vi "pulse data FFTfilter.vi"() -> ()   [LabVIEW 2016]
uses:
  <vilib>/Analysis/2dsp.llb/Real FFT.vi
  <vilib>/Analysis/2dsp.llb/Inverse Real FFT.vi
  <vilib>/Analysis/NI_AALPro.lvlib
panel:
  in  "lower cut off":dbl format="%.2f"
  in  "upper cut off":dbl=50000.0 format="%.2f"
  in  "filter":u16(ring) items=["Band Pass", "Band Stop"]
  in  "save interpolation?":bool
  in  "format":string="%f"
  in  "average traces?":u8=1 min=1 step=1
  in  "save plot?":bool
  in  "format":string="%f"
  out "plotted data":cluster{dbl[], dbl[]}(graph)
  in  "type of interpolation":u16(ring) items=["linear", "cubic spline", "polynomial"]
  in  "no. 1/B interpolation points":u16(ring) items=["1024", "2048", "4096", "8192", "16384", "32768"]
  in  "y domain":u16(ring) items=["channel A"]
  in  "x domain":u16(ring) items=["time (rising field)", "time (falling field)", "1/B (rising field)", "1/B (falling field)", "1/B (rising field + falling field)", "1/B (rising field - falling field)"]
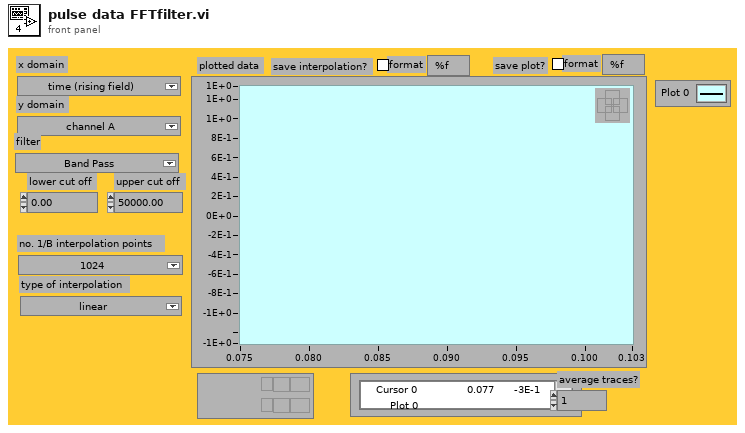
[diagram p1: front panel]
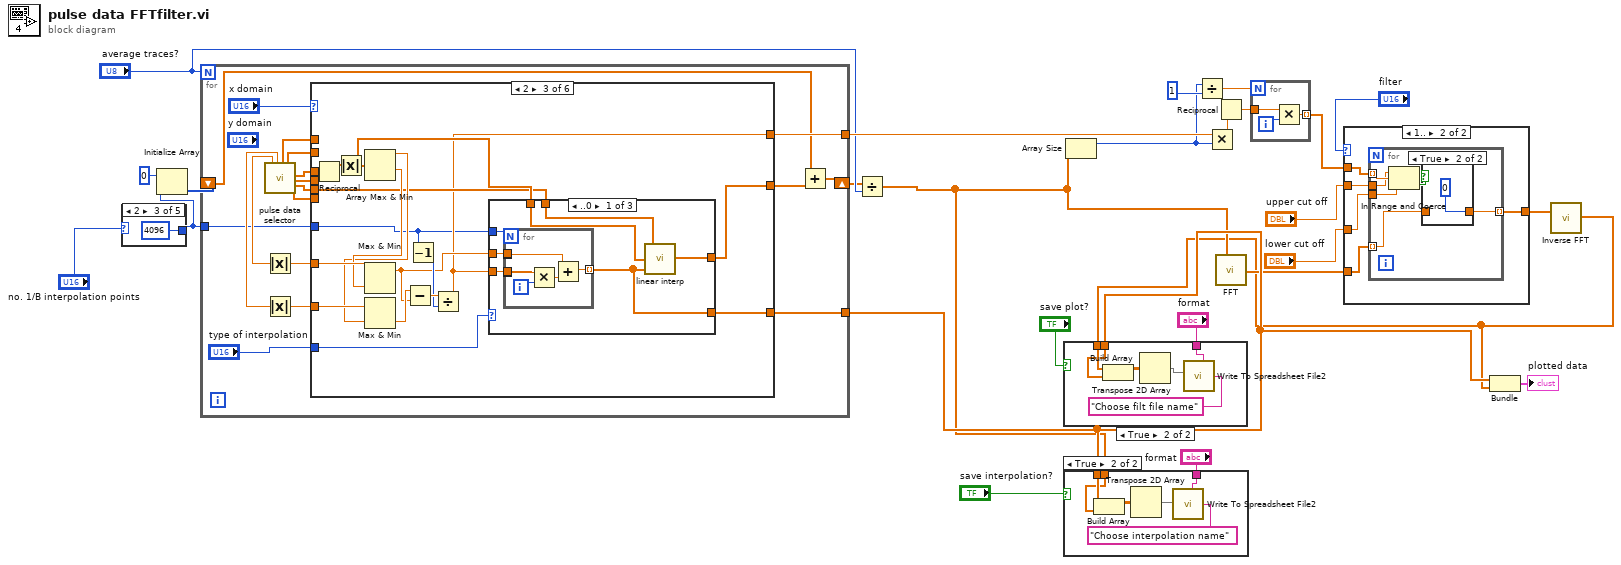
[diagram p0: block diagram]
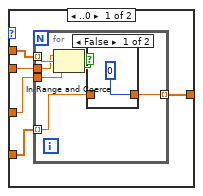
[diagram p2: hidden frame]
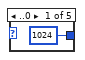
[diagram p6: hidden frame]
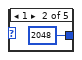
[diagram p7: hidden frame]
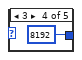
[diagram p8: hidden frame]
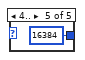
[diagram p9: hidden frame]
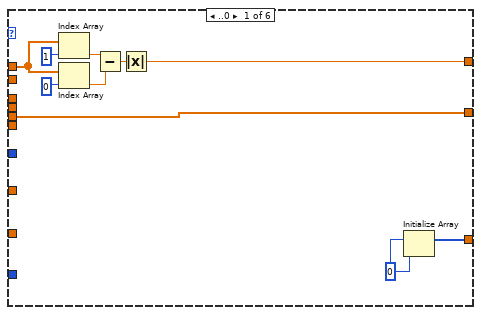
[diagram p10: hidden frame]
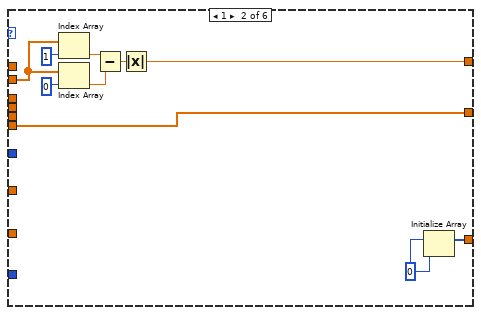
[diagram p11: hidden frame]
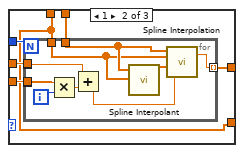
[diagram p12: hidden frame]
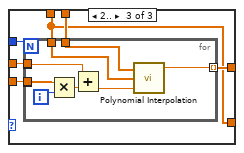
[diagram p13: hidden frame]
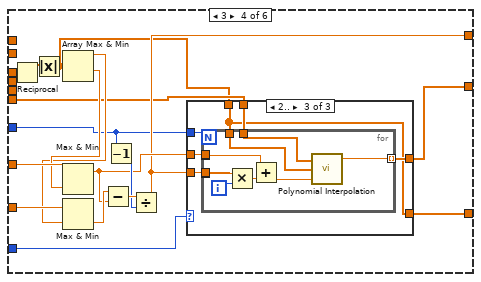
[diagram p14: hidden frame]
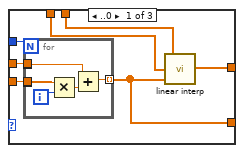
[diagram p15: hidden frame]
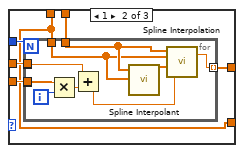
[diagram p16: hidden frame]
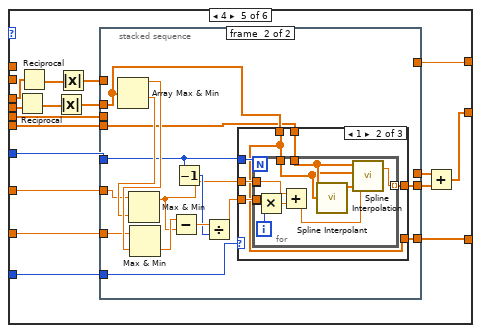
[diagram p17: hidden frame]
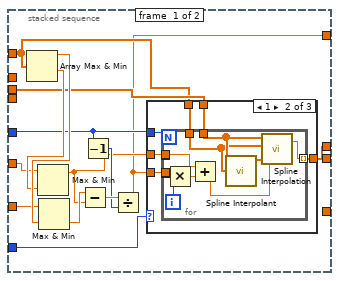
[diagram p18: hidden frame]
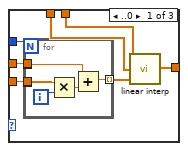
[diagram p19: hidden frame]
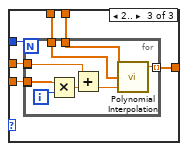
[diagram p20: hidden frame]
diagram:
  n1 = case shown="2" "no. 1/B interpolation points" {
    tunnel: [1024 2048 4096 8192 16384] -> w19
    frame ..0 {
    }
    frame 1 {
    }
    frame 2 {
    }
    frame 3 {
    }
    frame 4.. {
    }
  }
  n2 = Initialize Array(0, w19) -> (w18:i32[])
  n3 = for {
    N: "average traces?" -> [_]
    tunnel: w19 -> [w37]
    shift-right: [w33] -> w15
    shift-left: w18 -> [w35]
    tunnel: [w36] -> w17
    tunnel: [w32] -> w5
    n4 = call "pulse data selector.vi"() -> ("1/B start interpolation"=w43:dbl, "1/B end interpolation"=w44:dbl, "time rising"=w39:dbl[], "time falling"=w40:dbl[], "B rising"=w47:dbl[], "B falling"=w48:dbl[], "ch A rising"=w41:dbl[], "ch A falling"=w42:dbl[])  [unwired: 7 in, 5 out]
    n5 = Absolute Value(x=w43) -> (abs(x)=w45:dbl)
    n6 = Absolute Value(x=w44) -> (abs(x)=w46:dbl)
    n7 = case shown="2" "x domain" {
      tunnel: w39 -> [w57 _ _ _ _ _]
      tunnel: w40 -> [_ w63 _ _ _ _]
      tunnel: w41 -> [w53 _ w75 _ w196 w324]
      tunnel: w42 -> [_ w62 _ w132 w197 w325]
      tunnel: [w53 w62 w74 w135 w188 w316] -> w34
      tunnel: [w52 w64 w73 w134 w192 w320] -> w36
      tunnel: w37 -> [_ _ w71 w129 w187 w315]
      tunnel: w45 -> [_ _ w85 w144 w199 w327]
      tunnel: w46 -> [_ _ w83 w142 w198 w326]
      tunnel: w47 -> [_ _ w78 _ w194 w322]
      tunnel: w48 -> [_ _ _ w133 w201 w329]
      tunnel: "type of interpolation" -> [_ _ w77 w137 w200 w328]
      tunnel: [w50 w60 w70 w128 w186 w314] -> w32
      frame ..0 {
        w51 = 0
        n8 = Index Array(array=w57, index=1) -> (element=w56:dbl)
        n9 = Index Array(array=w57, index=0) -> (element=w55:dbl)
        n10 = Subtract(x=w56, y=w55) -> (x-y=w54:dbl)
        n11 = Absolute Value(x=w54) -> (abs(x)=w52:dbl)
        n12 = Initialize Array(w51, w51) -> (w50:i32[])
      }
      frame 1 {
        w61 = 0
        n13 = Index Array(array=w63, index=1) -> (element=w67:dbl)
        n14 = Index Array(array=w63, index=0) -> (element=w66:dbl)
        n15 = Subtract(x=w67, y=w66) -> (x-y=w65:dbl)
        n16 = Absolute Value(x=w65) -> (abs(x)=w64:dbl)
        n17 = Initialize Array(w61, w61) -> (w60:i32[])
      }
      frame 2 {
        n18 = Reciprocal(x=w78) -> (1/x=w72:dbl[])
        n19 = Absolute Value(x=w72) -> (abs(x)=w86:dbl[])
        n20 = Array Max & Min(array=w86) -> (max value=w82:dbl, min value=w84:dbl)  [unwired: 2 out]
        n21 = Max & Min(x=w85, y=w84) -> (max(x,y)=w76:dbl)  [unwired: 1 out]
        n22 = Max & Min(x=w83, y=w82) -> (min(x,y)=w81:dbl)  [unwired: 1 out]
        n23 = Subtract(x=w81, y=w76) -> (x-y=w80:dbl)
        n24 = Decrement(x=w71) -> (x-1=w79:i32)
        n25 = Divide(x=w80, y=w79) -> (x/y=w73:dbl)
        n26 = case shown="..0" w77 {
          tunnel: w71 -> [w93 w104 w119]
          tunnel: w76 -> [w92 w103 w118]
          tunnel: w73 -> [w91 w102 w117]
          tunnel: w86 -> [w89 w99 w114]
          tunnel: w75 -> [w90 w101 w116]
          tunnel: [w88 w100 w115] -> w74
          tunnel: [w87 w99 w114] -> w70
          frame ..0 {
            n27 = for {
              N: w93 -> [_]
              tunnel: [w95] -> _ mode=indexing
              tunnel: [w96] -> _ mode=indexing
              tunnel: w92 -> [w96]
              tunnel: w91 -> [w95]
              tunnel: [w94] -> w87 mode=indexing
              i -> [w98]
              n28 = Multiply(x=w95, y=w98) -> (x*y=w97:dbl)
              n29 = Add(x=w96, y=w97) -> (x+y=w94:dbl)
            }
            n30 = call "linear interp.vi"("x array"=w87, "X data"=w89, "Y data"=w90) -> ("y"=w88:dbl[])
          }
          frame 1 {
            n31 = for {
              N: w104 -> [_]
              tunnel: [w110] -> _ mode=indexing
              tunnel: [w111] -> _ mode=indexing
              tunnel: w103 -> [w111]
              tunnel: w102 -> [w110]
              tunnel: w99 -> [w105]
              tunnel: w101 -> [w109]
              tunnel: [w106] -> w100 mode=indexing
              i -> [w113]
              n32 = Multiply(x=w110, y=w113) -> (x*y=w112:dbl)
              n33 = Add(x=w111, y=w112) -> (x+y=w107:dbl)
              n34 = call <vilib>:"Spline Interpolant.vi"("X"=w105, "Y"=w109) -> ("Interpolant"=w108:dbl[])  [unwired: 2 in, 1 out]
              n35 = call <vilib>:"Spline Interpolation.vi"("x value"=w107, "Interpolant"=w108, "X"=w105, "Y"=w109) -> ("interpolation value"=w106:dbl)  [unwired: 1 out]
            }
          }
          frame 2.. {
            n36 = for {
              N: w119 -> [_]
              tunnel: [w124] -> _ mode=indexing
              tunnel: [w125] -> _ mode=indexing
              tunnel: w118 -> [w125]
              tunnel: w117 -> [w124]
              tunnel: w114 -> [w120]
              tunnel: w116 -> [w123]
              tunnel: [w121] -> w115 mode=indexing
              i -> [w127]
              n37 = Multiply(x=w124, y=w127) -> (x*y=w126:dbl)
              n38 = Add(x=w125, y=w126) -> (x+y=w122:dbl)
              n39 = call <vilib>:"Polynomial Interpolation.vi"("x value"=w122, "X"=w120, "Y"=w123) -> ("interpolation value"=w121:dbl)  [unwired: 2 out]
            }
          }
        }
      }
      frame 3 {
        n40 = Reciprocal(x=w133) -> (1/x=w131:dbl[])
        n41 = Absolute Value(x=w131) -> (abs(x)=w130:dbl[])
        n42 = Array Max & Min(array=w130) -> (max value=w141:dbl, min value=w143:dbl)  [unwired: 2 out]
        n43 = Max & Min(x=w144, y=w143) -> (max(x,y)=w136:dbl)  [unwired: 1 out]
        n44 = Max & Min(x=w142, y=w141) -> (min(x,y)=w140:dbl)  [unwired: 1 out]
        n45 = Subtract(x=w140, y=w136) -> (x-y=w139:dbl)
        n46 = Decrement(x=w129) -> (x-1=w138:i32)
        n47 = Divide(x=w139, y=w138) -> (x/y=w134:dbl)
        n48 = case shown="2.." w137 {
          tunnel: w129 -> [w151 w162 w177]
          tunnel: w136 -> [w150 w161 w176]
          tunnel: w134 -> [w149 w160 w175]
          tunnel: w130 -> [w147 w157 w172]
          tunnel: w132 -> [w148 w159 w174]
          tunnel: [w146 w158 w173] -> w135
          tunnel: [w145 w157 w172] -> w128
          frame ..0 {
            n49 = for {
              N: w151 -> [_]
              tunnel: [w153] -> _ mode=indexing
              tunnel: [w154] -> _ mode=indexing
              tunnel: w150 -> [w154]
              tunnel: w149 -> [w153]
              tunnel: [w152] -> w145 mode=indexing
              i -> [w156]
              n50 = Multiply(x=w153, y=w156) -> (x*y=w155:dbl)
              n51 = Add(x=w154, y=w155) -> (x+y=w152:dbl)
            }
            n52 = call "linear interp.vi"("x array"=w145, "X data"=w147, "Y data"=w148) -> ("y"=w146:dbl[])
          }
          frame 1 {
            n53 = for {
              N: w162 -> [_]
              tunnel: [w168] -> _ mode=indexing
              tunnel: [w169] -> _ mode=indexing
              tunnel: w161 -> [w169]
              tunnel: w160 -> [w168]
              tunnel: w157 -> [w166]
              tunnel: w159 -> [w167]
              tunnel: [w163] -> w158 mode=indexing
              i -> [w171]
              n54 = Multiply(x=w168, y=w171) -> (x*y=w170:dbl)
              n55 = Add(x=w169, y=w170) -> (x+y=w164:dbl)
              n56 = call <vilib>:"Spline Interpolant.vi"("X"=w166, "Y"=w167) -> ("Interpolant"=w165:dbl[])  [unwired: 2 in, 1 out]
              n57 = call <vilib>:"Spline Interpolation.vi"("x value"=w164, "Interpolant"=w165, "X"=w166, "Y"=w167) -> ("interpolation value"=w163:dbl)  [unwired: 1 out]
            }
          }
          frame 2.. {
            n58 = for {
              N: w177 -> [_]
              tunnel: [w182] -> _ mode=indexing
              tunnel: [w183] -> _ mode=indexing
              tunnel: w176 -> [w183]
              tunnel: w175 -> [w182]
              tunnel: w172 -> [w181]
              tunnel: w174 -> [w180]
              tunnel: [w178] -> w173 mode=indexing
              i -> [w185]
              n59 = Multiply(x=w182, y=w185) -> (x*y=w184:dbl)
              n60 = Add(x=w183, y=w184) -> (x+y=w179:dbl)
              n61 = call <vilib>:"Polynomial Interpolation.vi"("x value"=w179, "X"=w181, "Y"=w180) -> ("interpolation value"=w178:dbl)  [unwired: 2 out]
            }
          }
        }
      }
      frame 4 {
        n62 = Reciprocal(x=w201) -> (1/x=w202:dbl[])
        n63 = Reciprocal(x=w194) -> (1/x=w195:dbl[])
        n64 = Absolute Value(x=w202) -> (abs(x)=w191:dbl[])
        n65 = Absolute Value(x=w195) -> (abs(x)=w193:dbl[])
        n66 = stacked-sequence {
          tunnel: w200 -> [w204 w259]
          tunnel: w199 -> [w210 w266]
          tunnel: w198 -> [w209 w265]
          tunnel: w197 -> [_ w260]
          tunnel: w196 -> [w208 _]
          tunnel: w193 -> [w207 _]
          tunnel: w187 -> [w206 w264]
          tunnel: [_ w263] -> w190
          tunnel: [w203 _] -> w192
          tunnel: w191 -> [_ w261]
          tunnel: [w205 _] -> w189
          tunnel: [_ w258] -> w186
          frame #0 {
            n67 = Array Max & Min(array=w207) -> (max value=w212:dbl, min value=w211:dbl)  [unwired: 2 out]
            n68 = Max & Min(x=w210, y=w211) -> (max(x,y)=w213:dbl)  [unwired: 1 out]
            n69 = Max & Min(x=w209, y=w212) -> (min(x,y)=w214:dbl)  [unwired: 1 out]
            n70 = Subtract(x=w214, y=w213) -> (x-y=w216:dbl)
            n71 = Decrement(x=w206) -> (x-1=w215:i32)
            n72 = Divide(x=w216, y=w215) -> (x/y=w203:dbl)
            n73 = case shown="1" w204 {
              tunnel: w206 -> [w223 w234 w249]
              tunnel: w213 -> [w222 w233 w248]
              tunnel: w203 -> [w221 w232 w247]
              tunnel: w207 -> [w219 w231 w246]
              tunnel: w208 -> [w220 w230 w245]
              tunnel: [w217 w229 w244] -> w205
              frame ..0 {
                n74 = for {
                  N: w223 -> [_]
                  tunnel: [w225] -> _ mode=indexing
                  tunnel: [w226] -> _ mode=indexing
                  tunnel: w222 -> [w226]
                  tunnel: w221 -> [w225]
                  tunnel: [w224] -> w218 mode=indexing
                  i -> [w228]
                  n75 = Multiply(x=w225, y=w228) -> (x*y=w227:dbl)
                  n76 = Add(x=w226, y=w227) -> (x+y=w224:dbl)
                }
                n77 = call "linear interp.vi"("x array"=w218, "X data"=w219, "Y data"=w220) -> ("y"=w217:dbl[])
              }
              frame 1 {
                n78 = for {
                  N: w234 -> [_]
                  tunnel: [w240] -> _ mode=indexing
                  tunnel: [w241] -> _ mode=indexing
                  tunnel: w233 -> [w241]
                  tunnel: w232 -> [w240]
                  tunnel: w231 -> [w238]
                  tunnel: w230 -> [w239]
                  tunnel: [w235] -> w229 mode=indexing
                  i -> [w243]
                  n79 = Multiply(x=w240, y=w243) -> (x*y=w242:dbl)
                  n80 = Add(x=w241, y=w242) -> (x+y=w236:dbl)
                  n81 = call <vilib>:"Spline Interpolant.vi"("X"=w238, "Y"=w239) -> ("Interpolant"=w237:dbl[])  [unwired: 2 in, 1 out]
                  n82 = call <vilib>:"Spline Interpolation.vi"("x value"=w236, "Interpolant"=w237, "X"=w238, "Y"=w239) -> ("interpolation value"=w235:dbl)  [unwired: 1 out]
                }
              }
              frame 2.. {
                n83 = for {
                  N: w249 -> [_]
                  tunnel: [w254] -> _ mode=indexing
                  tunnel: [w255] -> _ mode=indexing
                  tunnel: w248 -> [w255]
                  tunnel: w247 -> [w254]
                  tunnel: w246 -> [w253]
                  tunnel: w245 -> [w252]
                  tunnel: [w250] -> w244 mode=indexing
                  i -> [w257]
                  n84 = Multiply(x=w254, y=w257) -> (x*y=w256:dbl)
                  n85 = Add(x=w255, y=w256) -> (x+y=w251:dbl)
                  n86 = call <vilib>:"Polynomial Interpolation.vi"("x value"=w251, "X"=w253, "Y"=w252) -> ("interpolation value"=w250:dbl)  [unwired: 2 out]
                }
              }
            }
          }
          frame #1 {
            n87 = Array Max & Min(array=w261) -> (max value=w268:dbl, min value=w267:dbl)  [unwired: 2 out]
            n88 = Max & Min(x=w266, y=w267) -> (max(x,y)=w269:dbl)  [unwired: 1 out]
            n89 = Max & Min(x=w265, y=w268) -> (min(x,y)=w270:dbl)  [unwired: 1 out]
            n90 = Subtract(x=w270, y=w269) -> (x-y=w272:dbl)
            n91 = Decrement(x=w264) -> (x-1=w271:i32)
            n92 = Divide(x=w272, y=w271) -> (x/y=w262:dbl)
            n93 = case shown="1" w259 {
              tunnel: w264 -> [w279 w290 w305]
              tunnel: w269 -> [w278 w289 w304]
              tunnel: w262 -> [w277 w288 w303]
              tunnel: w261 -> [w275 w285 w300]
              tunnel: w260 -> [w276 w287 w302]
              tunnel: [w274 w286 w301] -> w263
              tunnel: [w273 w285 w300] -> w258
              frame ..0 {
                n94 = for {
                  N: w279 -> [_]
                  tunnel: [w281] -> _ mode=indexing
                  tunnel: [w282] -> _ mode=indexing
                  tunnel: w278 -> [w282]
                  tunnel: w277 -> [w281]
                  tunnel: [w280] -> w273 mode=indexing
                  i -> [w284]
                  n95 = Multiply(x=w281, y=w284) -> (x*y=w283:dbl)
                  n96 = Add(x=w282, y=w283) -> (x+y=w280:dbl)
                }
                n97 = call "linear interp.vi"("x array"=w273, "X data"=w275, "Y data"=w276) -> ("y"=w274:dbl[])
              }
              frame 1 {
                n98 = for {
                  N: w290 -> [_]
                  tunnel: [w296] -> _ mode=indexing
                  tunnel: [w297] -> _ mode=indexing
                  tunnel: w289 -> [w297]
                  tunnel: w288 -> [w296]
                  tunnel: w285 -> [w294]
                  tunnel: w287 -> [w295]
                  tunnel: [w291] -> w286 mode=indexing
                  i -> [w299]
                  n99 = Multiply(x=w296, y=w299) -> (x*y=w298:dbl)
                  n100 = Add(x=w297, y=w298) -> (x+y=w292:dbl)
                  n101 = call <vilib>:"Spline Interpolant.vi"("X"=w294, "Y"=w295) -> ("Interpolant"=w293:dbl[])  [unwired: 2 in, 1 out]
                  n102 = call <vilib>:"Spline Interpolation.vi"("x value"=w292, "Interpolant"=w293, "X"=w294, "Y"=w295) -> ("interpolation value"=w291:dbl)  [unwired: 1 out]
                }
              }
              frame 2.. {
                n103 = for {
                  N: w305 -> [_]
                  tunnel: [w310] -> _ mode=indexing
                  tunnel: [w311] -> _ mode=indexing
                  tunnel: w304 -> [w311]
                  tunnel: w303 -> [w310]
                  tunnel: w300 -> [w309]
                  tunnel: w302 -> [w308]
                  tunnel: [w306] -> w301 mode=indexing
                  i -> [w313]
                  n104 = Multiply(x=w310, y=w313) -> (x*y=w312:dbl)
                  n105 = Add(x=w311, y=w312) -> (x+y=w307:dbl)
                  n106 = call <vilib>:"Polynomial Interpolation.vi"("x value"=w307, "X"=w309, "Y"=w308) -> ("interpolation value"=w306:dbl)  [unwired: 2 out]
                }
              }
            }
          }
        }
        n107 = Add(x=w189, y=w190) -> (x+y=w188:dbl[])
      }
      frame 5.. {
        n108 = Reciprocal(x=w329) -> (1/x=w330:dbl[])
        n109 = Reciprocal(x=w322) -> (1/x=w323:dbl[])
        n110 = Absolute Value(x=w330) -> (abs(x)=w319:dbl[])
        n111 = Absolute Value(x=w323) -> (abs(x)=w321:dbl[])
        n112 = stacked-sequence {
          tunnel: w328 -> [w331 w387]
          tunnel: w327 -> [w338 w394]
          tunnel: w326 -> [w337 w393]
          tunnel: w325 -> [_ w388]
          tunnel: w324 -> [w336 _]
          tunnel: w321 -> [w335 _]
          tunnel: w315 -> [w334 w392]
          tunnel: [_ w391] -> w318
          tunnel: [w332 _] -> w320
          tunnel: w319 -> [_ w389]
          tunnel: [w333 _] -> w317
          tunnel: [_ w386] -> w314
          frame #0 {
            n113 = Array Max & Min(array=w335) -> (max value=w340:dbl, min value=w339:dbl)  [unwired: 2 out]
            n114 = Max & Min(x=w338, y=w339) -> (max(x,y)=w341:dbl)  [unwired: 1 out]
            n115 = Max & Min(x=w337, y=w340) -> (min(x,y)=w342:dbl)  [unwired: 1 out]
            n116 = Subtract(x=w342, y=w341) -> (x-y=w344:dbl)
            n117 = Decrement(x=w334) -> (x-1=w343:i32)
            n118 = Divide(x=w344, y=w343) -> (x/y=w332:dbl)
            n119 = case shown="1" w331 {
              tunnel: w334 -> [w351 w362 w377]
              tunnel: w341 -> [w350 w361 w376]
              tunnel: w332 -> [w349 w360 w375]
              tunnel: w335 -> [w347 w359 w374]
              tunnel: w336 -> [w348 w358 w373]
              tunnel: [w345 w357 w372] -> w333
              frame ..0 {
                n120 = for {
                  N: w351 -> [_]
                  tunnel: [w353] -> _ mode=indexing
                  tunnel: [w354] -> _ mode=indexing
                  tunnel: w350 -> [w354]
                  tunnel: w349 -> [w353]
                  tunnel: [w352] -> w346 mode=indexing
                  i -> [w356]
                  n121 = Multiply(x=w353, y=w356) -> (x*y=w355:dbl)
                  n122 = Add(x=w354, y=w355) -> (x+y=w352:dbl)
                }
                n123 = call "linear interp.vi"("x array"=w346, "X data"=w347, "Y data"=w348) -> ("y"=w345:dbl[])
              }
              frame 1 {
                n124 = for {
                  N: w362 -> [_]
                  tunnel: [w368] -> _ mode=indexing
                  tunnel: [w369] -> _ mode=indexing
                  tunnel: w361 -> [w369]
                  tunnel: w360 -> [w368]
                  tunnel: w359 -> [w366]
                  tunnel: w358 -> [w367]
                  tunnel: [w363] -> w357 mode=indexing
                  i -> [w371]
                  n125 = Multiply(x=w368, y=w371) -> (x*y=w370:dbl)
                  n126 = Add(x=w369, y=w370) -> (x+y=w364:dbl)
                  n127 = call <vilib>:"Spline Interpolant.vi"("X"=w366, "Y"=w367) -> ("Interpolant"=w365:dbl[])  [unwired: 2 in, 1 out]
                  n128 = call <vilib>:"Spline Interpolation.vi"("x value"=w364, "Interpolant"=w365, "X"=w366, "Y"=w367) -> ("interpolation value"=w363:dbl)  [unwired: 1 out]
                }
              }
              frame 2.. {
                n129 = for {
                  N: w377 -> [_]
                  tunnel: [w382] -> _ mode=indexing
                  tunnel: [w383] -> _ mode=indexing
                  tunnel: w376 -> [w383]
                  tunnel: w375 -> [w382]
                  tunnel: w374 -> [w381]
                  tunnel: w373 -> [w380]
                  tunnel: [w378] -> w372 mode=indexing
                  i -> [w385]
                  n130 = Multiply(x=w382, y=w385) -> (x*y=w384:dbl)
                  n131 = Add(x=w383, y=w384) -> (x+y=w379:dbl)
                  n132 = call <vilib>:"Polynomial Interpolation.vi"("x value"=w379, "X"=w381, "Y"=w380) -> ("interpolation value"=w378:dbl)  [unwired: 2 out]
                }
              }
            }
          }
          frame #1 {
            n133 = Array Max & Min(array=w389) -> (max value=w396:dbl, min value=w395:dbl)  [unwired: 2 out]
            n134 = Max & Min(x=w394, y=w395) -> (max(x,y)=w397:dbl)  [unwired: 1 out]
            n135 = Max & Min(x=w393, y=w396) -> (min(x,y)=w398:dbl)  [unwired: 1 out]
            n136 = Subtract(x=w398, y=w397) -> (x-y=w400:dbl)
            n137 = Decrement(x=w392) -> (x-1=w399:i32)
            n138 = Divide(x=w400, y=w399) -> (x/y=w390:dbl)
            n139 = case shown="2.." w387 {
              tunnel: w392 -> [w407 w418 w433]
              tunnel: w397 -> [w406 w417 w432]
              tunnel: w390 -> [w405 w416 w431]
              tunnel: w389 -> [w403 w413 w428]
              tunnel: w388 -> [w404 w415 w430]
              tunnel: [w402 w414 w429] -> w391
              tunnel: [w401 w413 w428] -> w386
              frame ..0 {
                n140 = for {
                  N: w407 -> [_]
                  tunnel: [w409] -> _ mode=indexing
                  tunnel: [w410] -> _ mode=indexing
                  tunnel: w406 -> [w410]
                  tunnel: w405 -> [w409]
                  tunnel: [w408] -> w401 mode=indexing
                  i -> [w412]
                  n141 = Multiply(x=w409, y=w412) -> (x*y=w411:dbl)
                  n142 = Add(x=w410, y=w411) -> (x+y=w408:dbl)
                }
                n143 = call "linear interp.vi"("x array"=w401, "X data"=w403, "Y data"=w404) -> ("y"=w402:dbl[])
              }
              frame 1 {
                n144 = for {
                  N: w418 -> [_]
                  tunnel: [w424] -> _ mode=indexing
                  tunnel: [w425] -> _ mode=indexing
                  tunnel: w417 -> [w425]
                  tunnel: w416 -> [w424]
                  tunnel: w413 -> [w422]
                  tunnel: w415 -> [w423]
                  tunnel: [w419] -> w414 mode=indexing
                  i -> [w427]
                  n145 = Multiply(x=w424, y=w427) -> (x*y=w426:dbl)
                  n146 = Add(x=w425, y=w426) -> (x+y=w420:dbl)
                  n147 = call <vilib>:"Spline Interpolant.vi"("X"=w422, "Y"=w423) -> ("Interpolant"=w421:dbl[])  [unwired: 2 in, 1 out]
                  n148 = call <vilib>:"Spline Interpolation.vi"("x value"=w420, "Interpolant"=w421, "X"=w422, "Y"=w423) -> ("interpolation value"=w419:dbl)  [unwired: 1 out]
                }
              }
              frame 2.. {
                n149 = for {
                  N: w433 -> [_]
                  tunnel: [w438] -> _ mode=indexing
                  tunnel: [w439] -> _ mode=indexing
                  tunnel: w432 -> [w439]
                  tunnel: w431 -> [w438]
                  tunnel: w428 -> [w437]
                  tunnel: w430 -> [w436]
                  tunnel: [w434] -> w429 mode=indexing
                  i -> [w441]
                  n150 = Multiply(x=w438, y=w441) -> (x*y=w440:dbl)
                  n151 = Add(x=w439, y=w440) -> (x+y=w435:dbl)
                  n152 = call <vilib>:"Polynomial Interpolation.vi"("x value"=w435, "X"=w437, "Y"=w436) -> ("interpolation value"=w434:dbl)  [unwired: 2 out]
                }
              }
            }
          }
        }
        n153 = Subtract(x=w317, y=w318) -> (x-y=w316:dbl[])
      }
    }
    n154 = Add(x=w35, y=w34) -> (x+y=w33:dbl[])
  }
  n155 = Divide(x=w15, y="average traces?") -> (x/y=w3:dbl[])
  n156 = case shown="True" "save interpolation?" {
    tunnel: "format" -> [_ w445]
    tunnel: w5 -> [_ w444]
    tunnel: w3 -> [_ w443]
    frame False {
    }
    frame True {
      n157 = Build Array(w444, w443) -> (w447:dbl[][])
      n158 = Transpose 2D Array(2D array=w447) -> (transposed array=w446:dbl[][])
      n159 = call "Write To Spreadsheet File2.vi"("dialogue"="Choose interpolation name", "format (%.3f)"=w445, "2D data"=w446) -> ()  [unwired: 5 in, 1 out]
    }
  }
  n160 = Array Size(array=w3) -> (size(s)=w6:i32)
  n161 = Divide(x=w6, y=1) -> (x/y=w11:dbl)
  n162 = Multiply(x=w17, y=w6) -> (x*y=w26:dbl)
  n163 = Reciprocal(x=w26) -> (1/x=w12:dbl)
  n164 = call-poly <vilib>:"FFT.vi"("X"=w3) -> ("FFT {X}"=w4:cdb[])  [unwired: 9 in, 1 out]
  n165 = for {
    N: w11 -> [_]
    tunnel: w12 -> [w449]
    tunnel: [w448] -> w9 mode=indexing
    i -> [w450]
    n166 = Multiply(x=w449, y=w450) -> (x*y=w448:dbl)
  }
  n167 = case shown="1.." "filter" {
    tunnel: w9 -> [w455 w468]
    tunnel: "upper cut off" -> [w454 w467]
    tunnel: "lower cut off" -> [w453 w466]
    tunnel: w4 -> [w452 w465]
    tunnel: [w451 w464] -> w2
    frame ..0 {
      n168 = for {
        tunnel: w455 -> [w461] mode=indexing
        tunnel: w454 -> [w460]
        tunnel: w453 -> [w459]
        tunnel: w452 -> [w457] mode=indexing
        tunnel: [w456] -> w451 mode=indexing
        n169 = In Range and Coerce(upper limit=w460, x=w461, lower limit=w459) -> (In Range?=w458:bool)  [unwired: 1 out]
        n170 = case shown="False" w458 {
          tunnel: w457 -> [_ w463]
          tunnel: [0 w463] -> w456
          frame False {
          }
          frame True {
          }
        }
      }
    }
    frame 1.. {
      n171 = for {
        tunnel: w468 -> [w474] mode=indexing
        tunnel: w467 -> [w473]
        tunnel: w466 -> [w472]
        tunnel: w465 -> [w470] mode=indexing
        tunnel: [w469] -> w464 mode=indexing
        n172 = In Range and Coerce(upper limit=w473, x=w474, lower limit=w472) -> (In Range?=w471:bool)  [unwired: 1 out]
        n173 = case shown="True" w471 {
          tunnel: w470 -> [w475 _]
          tunnel: [w475 0] -> w469
          frame False {
          }
          frame True {
          }
        }
      }
    }
  }
  n174 = call-poly <vilib>:"Inverse FFT.vi"("FFT {X}"=w2) -> ("X"=w1:dbl[])  [unwired: 9 in, 1 out]
  n175 = case shown="True" "save plot?" {
    tunnel: "format" -> [_ w480]
    tunnel: w1 -> [_ w479]
    tunnel: w5 -> [_ w478]
    frame False {
    }
    frame True {
      n176 = Build Array(w479, w478) -> (w482:dbl[][])
      n177 = Transpose 2D Array(2D array=w482) -> (transposed array=w481:dbl[][])
      n178 = call "Write To Spreadsheet File2.vi"("dialogue"="Choose filt file name", "format (%.3f)"=w480, "2D data"=w481) -> ()  [unwired: 5 in, 1 out]
    }
  }
  n179 = Bundle(w5, "X"=w1) -> (→"plotted data":cluster{dbl[], "X":dbl[]})  [unwired: 1 in]
